vi "DialogCfg.vi"(8 "error in (no error)":errorcluster, 11 "Sequence in":refnum<class "Sequence.lvclass">) -> (0 "error out":errorcluster, 1 "Cancelled?":bool, 3 "Sequence out":refnum<class "Sequence.lvclass">, 4 "TestSequence":T1[](array[typedef]))   [LabVIEW 2017]
uses:
  SequenceSubvis/PolarizationSelect.ctl
  SequenceSubvis/RF Direction.ctl
  Sequence.lvclass
  SequenceSubvis/TestStepTypes.ctl
  SequenceSubvis/TestStep-StepType.ctl
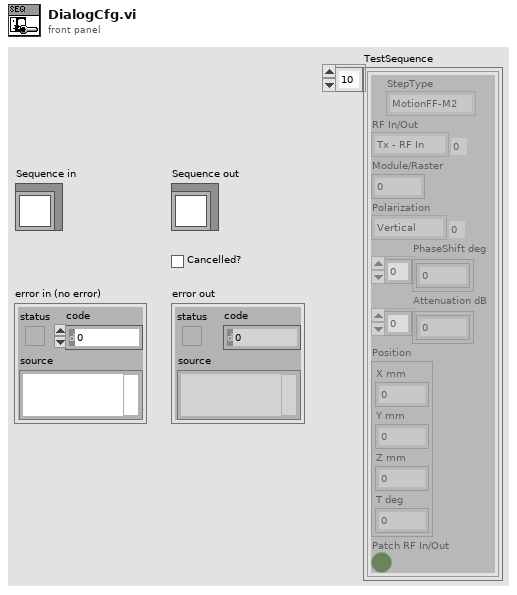
[diagram p1: front panel]
types:
  T1 = typedef "TestStep-StepType.ctl" = cluster{"StepType":T2, "RF In/Out":T3, "Module/Raster":i32, "Polarization":T4, "PhaseShift deg":dbl[], "Attenuation dB":dbl[], "Position":cluster{"X mm":dbl, "Y mm":dbl, "Z mm":dbl, "T deg":dbl}, "Patch RF In/Out":bool}
  T2 = typedef "TestStepTypes.ctl" = enum16{"MotionFF-M2", "Motion", "SweepTest", "RasterTest", "Finish", "64ModuleCfg"}
  T3 = typedef "RF Direction.ctl" = enum16{"Tx - RF In", "Rx - RF Out"}
  T4 = typedef "PolarizationSelect.ctl" = enum16{"Vertical", "Horizontal"}
  T5 = cluster{"StepType":enum16{"Patch", "Motion", "SweepTest", "RasterTest", "Finish"}, "RF In/Out":T3, "Module/Raster":i32, "Polarization":T4, "PhaseShift deg":dbl[], "Attenuation dB":dbl[], "Position":cluster{"X mm":dbl, "Y mm":dbl, "Z mm":dbl, "T deg":dbl}, "Patch RF In/Out":bool}[]
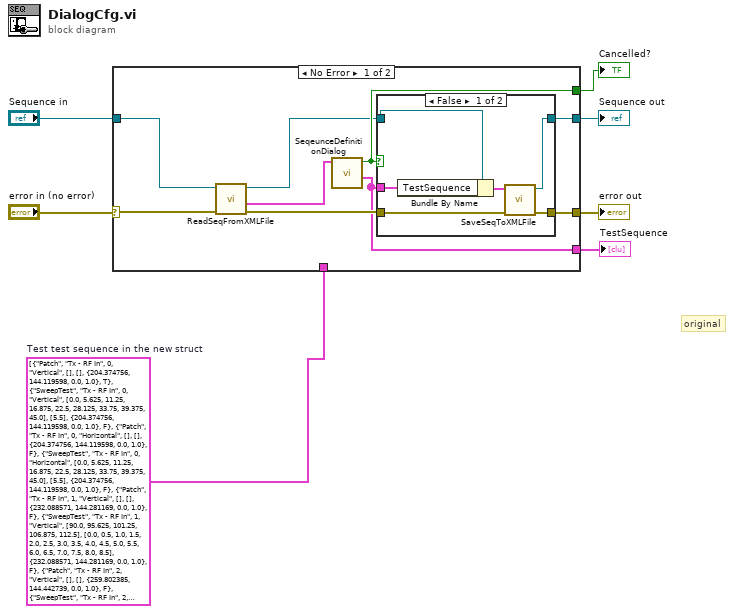
[diagram p0: block diagram]
diagram:
  w1 = T5 [{"StepType"=enum."Patch", "RF In/Out"=enum."Tx - RF In", "Module/Raster"=0, "Polarization"=enum."Vertical", "PhaseShift deg"=[], "Attenuation dB"=[], "Position"={"X mm"=204.374756, "Y mm"=144.119598, "Z mm"=0.0, "T deg"=1.0}, "Patch RF In/Out"=TRUE}, {"StepType"=enum."SweepTest", "RF In/Out"=enum."Tx - RF In", "Module/Raster"=0, "Polarization"=enum."Vertical", "PhaseShift deg"=[0.0, 5.625, 11.25, 16.875, 22.5, 28.125, 33.75, 39.375, 45.0], "Attenuation dB"=[5.5], "Position"={"X mm"=204.374756, "Y mm"=144.119598, "Z mm"=0.0, "T deg"=1.0}, "Patch RF In/Out"=FALSE}, {"StepType"=enum."Patch", "RF In/Out"=enum."Tx - RF In", "Module/Raster"=0, "Polarization"=enum."Horizontal", "PhaseShift deg"=[], "Attenuation dB"=[], "Position"={"X mm"=204.374756, "Y mm"=144.119598, "Z mm"=0.0, "T deg"=1.0}, "Patch RF In/Out"=FALSE}, {"StepType"=enum."SweepTest", "RF In/Out"=enum."Tx - RF In", "Module/Raster"=0, "Polarization"=enum."Horizontal", "PhaseShift deg"=[0.0, 5.625, 11.25, 16.875, 22.5, 28.125, 33.75, 39.375, 45.0], "Attenuation dB"=[5.5], "Position"={"X mm"=204.374756, "Y mm"=144.119598, "Z mm"=0.0, "T deg"=1.0}, "Patch RF In/Out"=FALSE}, {"StepType"=enum."Patch", "RF In/Out"=enum."Tx - RF In", "Module/Raster"=1, "Polarization"=enum."Vertical", "PhaseShift deg"=[], "Attenuation dB"=[], "Position"={"X mm"=232.088571, "Y mm"=144.281169, "Z mm"=0.0, "T deg"=1.0}, "Patch RF In/Out"=FALSE}, {"StepType"=enum."SweepTest", "RF In/Out"=enum."Tx - RF In", "Module/Raster"=1, "Polarization"=enum."Vertical", "PhaseShift deg"=[90.0, 95.625, 101.25, 106.875, 112.5], "Attenuation dB"=[0.0, 0.5, 1.0, 1.5, 2.0, 2.5, 3.0, 3.5, 4.0, 4.5, 5.0, 5.5, 6.0, 6.5, 7.0, 7.5, 8.0, 8.5], "Position"={"X mm"=232.088571, "Y mm"=144.281169, "Z mm"=0.0, "T deg"=1.0}, "Patch RF In/Out"=FALSE}, {"StepType"=enum."Patch", "RF In/Out"=enum."Tx - RF In", "Module/Raster"=2, "Polarization"=enum."Vertical", "PhaseShift deg"=[], "Attenuation dB"=[], "Position"={"X mm"=259.802385, "Y mm"=144.442739, "Z mm"=0.0, "T deg"=1.0}, "Patch RF In/Out"=FALSE}, {"StepType"=enum."SweepTest", "RF In/Out"=enum."Tx - RF In", "Module/Raster"=2, "Polarization"=enum."Vertical", "PhaseShift deg"=[11.25, 16.875, 22.5, 28.125, 33.75, 39.375, 45.0, 50.625, 56.25, 61.875, 67.5, 73.125, 78.75, 84.375, 90.0, 95.625, 101.25, 106.875, 112.5], "Attenuation dB"=[0.0, 5.5, 7.0, 8.0, 9.0, 9.5], "Position"={"X mm"=259.802385, "Y mm"=144.442739, "Z mm"=0.0, "T deg"=1.0}, "Patch RF In/Out"=FALSE}, {"StepType"=enum."Patch", "RF In/Out"=enum."Tx - RF In", "Module/Raster"=15, "Polarization"=enum."Vertical", "PhaseShift deg"=[], "Attenuation dB"=[], "Position"={"X mm"=398.209889, "Y mm"=172.964406, "Z mm"=0.0, "T deg"=1.0}, "Patch RF In/Out"=FALSE}, {"StepType"=enum."SweepTest", "RF In/Out"=enum."Tx - RF In", "Module/Raster"=15, "Polarization"=enum."Vertical", "PhaseShift deg"=[0.0, 5.625, 11.25, 16.875, 22.5], "Attenuation dB"=[0.0, 0.5, 1.0, 1.5, 2.0], "Position"={"X mm"=398.209889, "Y mm"=172.964406, "Z mm"=0.0, "T deg"=1.0}, "Patch RF In/Out"=FALSE}, {"StepType"=enum."Patch", "RF In/Out"=enum."Tx - RF In", "Module/Raster"=17, "Polarization"=enum."Vertical", "PhaseShift deg"=[], "Attenuation dB"=[], "Position"={"X mm"=231.76543, "Y mm"=199.708798, "Z mm"=0.0, "T deg"=1.0}, "Patch RF In/Out"=FALSE}, {"StepType"=enum."SweepTest", "RF In/Out"=enum."Tx - RF In", "Module/Raster"=17, "Polarization"=enum."Vertical", "PhaseShift deg"=[0.0, 5.625], "Attenuation dB"=[0.0, 0.5], "Position"={"X mm"=231.76543, "Y mm"=199.708798, "Z mm"=0.0, "T deg"=1.0}, "Patch RF In/Out"=FALSE}, {"StepType"=enum."Patch", "RF In/Out"=enum."Tx - RF In", "Module/Raster"=21, "Polarization"=enum."Vertical", "PhaseShift deg"=[], "Attenuation dB"=[], "Position"={"X mm"=342.620689, "Y mm"=200.35508, "Z mm"=0.0, "T deg"=1.0}, "Patch RF In/Out"=FALSE}, {"StepType"=enum."SweepTest", "RF In/Out"=enum."Tx - RF In", "Module/Raster"=21, "Polarization"=enum."Vertical", "PhaseShift deg"=[0.0], "Attenuation dB"=[0.0], "Position"={"X mm"=342.620689, "Y mm"=200.35508, "Z mm"=0.0, "T deg"=1.0}, "Patch RF In/Out"=FALSE}, {"StepType"=enum."Patch", "RF In/Out"=enum."Tx - RF In", "Module/Raster"=23, "Polarization"=enum."Vertical", "PhaseShift deg"=[], "Attenuation dB"=[], "Position"={"X mm"=398.048318, "Y mm"=200.678221, "Z mm"=0.0, "T deg"=1.0}, "Patch RF In/Out"=FALSE}, {"StepType"=enum."SweepTest", "RF In/Out"=enum."Tx - RF In", "Module/Raster"=23, "Polarization"=enum."Vertical", "PhaseShift deg"=[0.0], "Attenuation dB"=[0.0], "Position"={"X mm"=398.048318, "Y mm"=200.678221, "Z mm"=0.0, "T deg"=1.0}, "Patch RF In/Out"=FALSE}, {"StepType"=enum."Patch", "RF In/Out"=enum."Tx - RF In", "Module/Raster"=24, "Polarization"=enum."Vertical", "PhaseShift deg"=[], "Attenuation dB"=[], "Position"={"X mm"=203.890045, "Y mm"=227.261043, "Z mm"=0.0, "T deg"=1.0}, "Patch RF In/Out"=FALSE}, {"StepType"=enum."SweepTest", "RF In/Out"=enum."Tx - RF In", "Module/Raster"=24, "Polarization"=enum."Vertical", "PhaseShift deg"=[0.0, 5.625, 11.25], "Attenuation dB"=[0.0], "Position"={"X mm"=203.890045, "Y mm"=227.261043, "Z mm"=0.0, "T deg"=1.0}, "Patch RF In/Out"=FALSE}, {"StepType"=enum."Patch", "RF In/Out"=enum."Tx - RF In", "Module/Raster"=25, "Polarization"=enum."Vertical", "PhaseShift deg"=[], "Attenuation dB"=[], "Position"={"X mm"=231.603859, "Y mm"=227.422613, "Z mm"=0.0, "T deg"=1.0}, "Patch RF In/Out"=FALSE}, {"StepType"=enum."SweepTest", "RF In/Out"=enum."Tx - RF In", "Module/Raster"=25, "Polarization"=enum."Vertical", "PhaseShift deg"=[0.0], "Attenuation dB"=[0.0], "Position"={"X mm"=231.603859, "Y mm"=227.422613, "Z mm"=0.0, "T deg"=1.0}, "Patch RF In/Out"=FALSE}, {"StepType"=enum."Patch", "RF In/Out"=enum."Tx - RF In", "Module/Raster"=31, "Polarization"=enum."Vertical", "PhaseShift deg"=[], "Attenuation dB"=[], "Position"={"X mm"=397.886748, "Y mm"=228.392036, "Z mm"=0.0, "T deg"=1.0}, "Patch RF In/Out"=FALSE}, {"StepType"=enum."SweepTest", "RF In/Out"=enum."Tx - RF In", "Module/Raster"=31, "Polarization"=enum."Vertical", "PhaseShift deg"=[0.0, 5.625], "Attenuation dB"=[0.0], "Position"={"X mm"=397.886748, "Y mm"=228.392036, "Z mm"=0.0, "T deg"=1.0}, "Patch RF In/Out"=FALSE}, {"StepType"=enum."Patch", "RF In/Out"=enum."Tx - RF In", "Module/Raster"=31, "Polarization"=enum."Horizontal", "PhaseShift deg"=[], "Attenuation dB"=[], "Position"={"X mm"=397.886748, "Y mm"=228.392036, "Z mm"=0.0, "T deg"=1.0}, "Patch RF In/Out"=FALSE}, {"StepType"=enum."SweepTest", "RF In/Out"=enum."Tx - RF In", "Module/Raster"=31, "Polarization"=enum."Horizontal", "PhaseShift deg"=[0.0, 5.625], "Attenuation dB"=[0.0], "Position"={"X mm"=397.886748, "Y mm"=228.392036, "Z mm"=0.0, "T deg"=1.0}, "Patch RF In/Out"=FALSE}, {"StepType"=enum."Patch", "RF In/Out"=enum."Tx - RF In", "Module/Raster"=39, "Polarization"=enum."Vertical", "PhaseShift deg"=[], "Attenuation dB"=[], "Position"={"X mm"=397.725177, "Y mm"=256.10585, "Z mm"=0.0, "T deg"=1.0}, "Patch RF In/Out"=FALSE}, {"StepType"=enum."SweepTest", "RF In/Out"=enum."Tx - RF In", "Module/Raster"=39, "Polarization"=enum."Vertical", "PhaseShift deg"=[0.0], "Attenuation dB"=[0.0], "Position"={"X mm"=397.725177, "Y mm"=256.10585, "Z mm"=0.0, "T deg"=1.0}, "Patch RF In/Out"=FALSE}, {"StepType"=enum."Patch", "RF In/Out"=enum."Tx - RF In", "Module/Raster"=44, "Polarization"=enum."Vertical", "PhaseShift deg"=[], "Attenuation dB"=[], "Position"={"X mm"=314.422163, "Y mm"=283.334954, "Z mm"=0.0, "T deg"=1.0}, "Patch RF In/Out"=FALSE}, {"StepType"=enum."SweepTest", "RF In/Out"=enum."Tx - RF In", "Module/Raster"=44, "Polarization"=enum."Vertical", "PhaseShift deg"=[0.0, 5.625], "Attenuation dB"=[0.0, 0.5], "Position"={"X mm"=314.422163, "Y mm"=283.334954, "Z mm"=0.0, "T deg"=1.0}, "Patch RF In/Out"=FALSE}, {"StepType"=enum."Patch", "RF In/Out"=enum."Tx - RF In", "Module/Raster"=45, "Polarization"=enum."Vertical", "PhaseShift deg"=[], "Attenuation dB"=[], "Position"={"X mm"=342.135977, "Y mm"=283.496524, "Z mm"=0.0, "T deg"=1.0}, "Patch RF In/Out"=FALSE}, {"StepType"=enum."SweepTest", "RF In/Out"=enum."Tx - RF In", "Module/Raster"=45, "Polarization"=enum."Vertical", "PhaseShift deg"=[0.0], "Attenuation dB"=[0.0], "Position"={"X mm"=342.135977, "Y mm"=283.496524, "Z mm"=0.0, "T deg"=1.0}, "Patch RF In/Out"=FALSE}, {"StepType"=enum."Patch", "RF In/Out"=enum."Tx - RF In", "Module/Raster"=46, "Polarization"=enum."Vertical", "PhaseShift deg"=[], "Attenuation dB"=[], "Position"={"X mm"=369.849792, "Y mm"=283.658095, "Z mm"=0.0, "T deg"=1.0}, "Patch RF In/Out"=FALSE}, {"StepType"=enum."SweepTest", "RF In/Out"=enum."Tx - RF In", "Module/Raster"=46, "Polarization"=enum."Vertical", "PhaseShift deg"=[0.0, 5.625], "Attenuation dB"=[0.0, 0.5], "Position"={"X mm"=369.849792, "Y mm"=283.658095, "Z mm"=0.0, "T deg"=1.0}, "Patch RF In/Out"=FALSE}, {"StepType"=enum."Patch", "RF In/Out"=enum."Tx - RF In", "Module/Raster"=47, "Polarization"=enum."Vertical", "PhaseShift deg"=[], "Attenuation dB"=[], "Position"={"X mm"=397.563607, "Y mm"=283.819665, "Z mm"=0.0, "T deg"=1.0}, "Patch RF In/Out"=FALSE}, {"StepType"=enum."SweepTest", "RF In/Out"=enum."Tx - RF In", "Module/Raster"=47, "Polarization"=enum."Vertical", "PhaseShift deg"=[0.0], "Attenuation dB"=[0.0], "Position"={"X mm"=397.563607, "Y mm"=283.819665, "Z mm"=0.0, "T deg"=1.0}, "Patch RF In/Out"=FALSE}, {"StepType"=enum."Patch", "RF In/Out"=enum."Tx - RF In", "Module/Raster"=48, "Polarization"=enum."Vertical", "PhaseShift deg"=[], "Attenuation dB"=[], "Position"={"X mm"=203.405333, "Y mm"=310.402487, "Z mm"=0.0, "T deg"=1.0}, "Patch RF In/Out"=FALSE}, {"StepType"=enum."SweepTest", "RF In/Out"=enum."Tx - RF In", "Module/Raster"=48, "Polarization"=enum."Vertical", "PhaseShift deg"=[28.125], "Attenuation dB"=[2.5], "Position"={"X mm"=203.405333, "Y mm"=310.402487, "Z mm"=0.0, "T deg"=1.0}, "Patch RF In/Out"=FALSE}, {"StepType"=enum."Patch", "RF In/Out"=enum."Tx - RF In", "Module/Raster"=48, "Polarization"=enum."Horizontal", "PhaseShift deg"=[], "Attenuation dB"=[], "Position"={"X mm"=203.405333, "Y mm"=310.402487, "Z mm"=0.0, "T deg"=1.0}, "Patch RF In/Out"=FALSE}, {"StepType"=enum."SweepTest", "RF In/Out"=enum."Tx - RF In", "Module/Raster"=48, "Polarization"=enum."Horizontal", "PhaseShift deg"=[28.125], "Attenuation dB"=[2.5], "Position"={"X mm"=203.405333, "Y mm"=310.402487, "Z mm"=0.0, "T deg"=1.0}, "Patch RF In/Out"=FALSE}, {"StepType"=enum."Patch", "RF In/Out"=enum."Tx - RF In", "Module/Raster"=55, "Polarization"=enum."Vertical", "PhaseShift deg"=[], "Attenuation dB"=[], "Position"={"X mm"=397.402037, "Y mm"=311.53348, "Z mm"=0.0, "T deg"=1.0}, "Patch RF In/Out"=FALSE}, {"StepType"=enum."SweepTest", "RF In/Out"=enum."Tx - RF In", "Module/Raster"=55, "Polarization"=enum."Vertical", "PhaseShift deg"=[0.0, 5.625, 11.25, 16.875, 22.5], "Attenuation dB"=[0.0, 0.5, 1.0], "Position"={"X mm"=397.402037, "Y mm"=311.53348, "Z mm"=0.0, "T deg"=1.0}, "Patch RF In/Out"=FALSE}, {"StepType"=enum."Patch", "RF In/Out"=enum."Tx - RF In", "Module/Raster"=59, "Polarization"=enum."Vertical", "PhaseShift deg"=[], "Attenuation dB"=[], "Position"={"X mm"=286.385207, "Y mm"=338.601013, "Z mm"=0.0, "T deg"=1.0}, "Patch RF In/Out"=FALSE}, {"StepType"=enum."SweepTest", "RF In/Out"=enum."Tx - RF In", "Module/Raster"=59, "Polarization"=enum."Vertical", "PhaseShift deg"=[0.0], "Attenuation dB"=[0.0], "Position"={"X mm"=286.385207, "Y mm"=338.601013, "Z mm"=0.0, "T deg"=1.0}, "Patch RF In/Out"=FALSE}, {"StepType"=enum."Patch", "RF In/Out"=enum."Tx - RF In", "Module/Raster"=59, "Polarization"=enum."Horizontal", "PhaseShift deg"=[], "Attenuation dB"=[], "Position"={"X mm"=286.385207, "Y mm"=338.601013, "Z mm"=0.0, "T deg"=1.0}, "Patch RF In/Out"=FALSE}, {"StepType"=enum."SweepTest", "RF In/Out"=enum."Tx - RF In", "Module/Raster"=59, "Polarization"=enum."Horizontal", "PhaseShift deg"=[0.0], "Attenuation dB"=[0.0], "Position"={"X mm"=286.385207, "Y mm"=338.601013, "Z mm"=0.0, "T deg"=1.0}, "Patch RF In/Out"=FALSE}, {"StepType"=enum."Patch", "RF In/Out"=enum."Tx - RF In", "Module/Raster"=62, "Polarization"=enum."Vertical", "PhaseShift deg"=[], "Attenuation dB"=[], "Position"={"X mm"=369.526651, "Y mm"=339.085724, "Z mm"=0.0, "T deg"=1.0}, "Patch RF In/Out"=FALSE}, {"StepType"=enum."SweepTest", "RF In/Out"=enum."Tx - RF In", "Module/Raster"=62, "Polarization"=enum."Vertical", "PhaseShift deg"=[0.0, 5.625, 11.25, 16.875, 22.5, 28.125], "Attenuation dB"=[0.0, 0.5, 1.0, 1.5, 2.0, 2.5], "Position"={"X mm"=369.526651, "Y mm"=339.085724, "Z mm"=0.0, "T deg"=1.0}, "Patch RF In/Out"=FALSE}, {"StepType"=enum."Patch", "RF In/Out"=enum."Tx - RF In", "Module/Raster"=63, "Polarization"=enum."Vertical", "PhaseShift deg"=[], "Attenuation dB"=[], "Position"={"X mm"=397.240466, "Y mm"=339.247295, "Z mm"=0.0, "T deg"=1.0}, "Patch RF In/Out"=FALSE}, {"StepType"=enum."SweepTest", "RF In/Out"=enum."Tx - RF In", "Module/Raster"=63, "Polarization"=enum."Vertical", "PhaseShift deg"=[0.0, 5.625, 11.25, 16.875, 22.5, 28.125], "Attenuation dB"=[0.0, 0.5, 1.0, 1.5, 2.0, 2.5], "Position"={"X mm"=397.240466, "Y mm"=339.247295, "Z mm"=0.0, "T deg"=1.0}, "Patch RF In/Out"=FALSE}, {"StepType"=enum."Patch", "RF In/Out"=enum."Rx - RF Out", "Module/Raster"=0, "Polarization"=enum."Vertical", "PhaseShift deg"=[], "Attenuation dB"=[], "Position"={"X mm"=204.374756, "Y mm"=144.119598, "Z mm"=0.0, "T deg"=1.0}, "Patch RF In/Out"=TRUE}, {"StepType"=enum."SweepTest", "RF In/Out"=enum."Rx - RF Out", "Module/Raster"=0, "Polarization"=enum."Vertical", "PhaseShift deg"=[0.0, 5.625, 11.25, 16.875, 22.5, 28.125, 33.75, 39.375, 45.0], "Attenuation dB"=[5.5], "Position"={"X mm"=204.374756, "Y mm"=144.119598, "Z mm"=0.0, "T deg"=1.0}, "Patch RF In/Out"=FALSE}, {"StepType"=enum."Patch", "RF In/Out"=enum."Rx - RF Out", "Module/Raster"=0, "Polarization"=enum."Horizontal", "PhaseShift deg"=[], "Attenuation dB"=[], "Position"={"X mm"=204.374756, "Y mm"=144.119598, "Z mm"=0.0, "T deg"=1.0}, "Patch RF In/Out"=FALSE}, {"StepType"=enum."SweepTest", "RF In/Out"=enum."Rx - RF Out", "Module/Raster"=0, "Polarization"=enum."Horizontal", "PhaseShift deg"=[0.0, 5.625, 11.25, 16.875, 22.5, 28.125, 33.75, 39.375, 45.0], "Attenuation dB"=[5.5], "Position"={"X mm"=204.374756, "Y mm"=144.119598, "Z mm"=0.0, "T deg"=1.0}, "Patch RF In/Out"=FALSE}, {"StepType"=enum."Patch", "RF In/Out"=enum."Rx - RF Out", "Module/Raster"=17, "Polarization"=enum."Horizontal", "PhaseShift deg"=[], "Attenuation dB"=[], "Position"={"X mm"=231.76543, "Y mm"=199.708798, "Z mm"=0.0, "T deg"=1.0}, "Patch RF In/Out"=FALSE}, {"StepType"=enum."SweepTest", "RF In/Out"=enum."Rx - RF Out", "Module/Raster"=17, "Polarization"=enum."Horizontal", "PhaseShift deg"=[0.0, 5.625], "Attenuation dB"=[0.0, 0.5], "Position"={"X mm"=231.76543, "Y mm"=199.708798, "Z mm"=0.0, "T deg"=1.0}, "Patch RF In/Out"=FALSE}, {"StepType"=enum."Patch", "RF In/Out"=enum."Rx - RF Out", "Module/Raster"=28, "Polarization"=enum."Vertical", "PhaseShift deg"=[], "Attenuation dB"=[], "Position"={"X mm"=314.745304, "Y mm"=227.907324, "Z mm"=0.0, "T deg"=1.0}, "Patch RF In/Out"=FALSE}, {"StepType"=enum."SweepTest", "RF In/Out"=enum."Rx - RF Out", "Module/Raster"=28, "Polarization"=enum."Vertical", "PhaseShift deg"=[0.0], "Attenuation dB"=[0.0], "Position"={"X mm"=314.745304, "Y mm"=227.907324, "Z mm"=0.0, "T deg"=1.0}, "Patch RF In/Out"=FALSE}, {"StepType"=enum."Patch", "RF In/Out"=enum."Rx - RF Out", "Module/Raster"=28, "Polarization"=enum."Horizontal", "PhaseShift deg"=[], "Attenuation dB"=[], "Position"={"X mm"=314.745304, "Y mm"=227.907324, "Z mm"=0.0, "T deg"=1.0}, "Patch RF In/Out"=FALSE}, {"StepType"=enum."SweepTest", "RF In/Out"=enum."Rx - RF Out", "Module/Raster"=28, "Polarization"=enum."Horizontal", "PhaseShift deg"=[0.0], "Attenuation dB"=[0.0], "Position"={"X mm"=314.745304, "Y mm"=227.907324, "Z mm"=0.0, "T deg"=1.0}, "Patch RF In/Out"=FALSE}, {"StepType"=enum."Patch", "RF In/Out"=enum."Rx - RF Out", "Module/Raster"=31, "Polarization"=enum."Vertical", "PhaseShift deg"=[], "Attenuation dB"=[], "Position"={"X mm"=397.886748, "Y mm"=228.392036, "Z mm"=0.0, "T deg"=1.0}, "Patch RF In/Out"=FALSE}, {"StepType"=enum."SweepTest", "RF In/Out"=enum."Rx - RF Out", "Module/Raster"=31, "Polarization"=enum."Vertical", "PhaseShift deg"=[0.0, 5.625], "Attenuation dB"=[0.0], "Position"={"X mm"=397.886748, "Y mm"=228.392036, "Z mm"=0.0, "T deg"=1.0}, "Patch RF In/Out"=FALSE}, {"StepType"=enum."Patch", "RF In/Out"=enum."Rx - RF Out", "Module/Raster"=31, "Polarization"=enum."Horizontal", "PhaseShift deg"=[], "Attenuation dB"=[], "Position"={"X mm"=397.886748, "Y mm"=228.392036, "Z mm"=0.0, "T deg"=1.0}, "Patch RF In/Out"=FALSE}, {"StepType"=enum."SweepTest", "RF In/Out"=enum."Rx - RF Out", "Module/Raster"=31, "Polarization"=enum."Horizontal", "PhaseShift deg"=[0.0, 5.625], "Attenuation dB"=[0.0], "Position"={"X mm"=397.886748, "Y mm"=228.392036, "Z mm"=0.0, "T deg"=1.0}, "Patch RF In/Out"=FALSE}, {"StepType"=enum."Patch", "RF In/Out"=enum."Rx - RF Out", "Module/Raster"=36, "Polarization"=enum."Vertical", "PhaseShift deg"=[], "Attenuation dB"=[], "Position"={"X mm"=314.583733, "Y mm"=255.621139, "Z mm"=0.0, "T deg"=1.0}, "Patch RF In/Out"=FALSE}, {"StepType"=enum."SweepTest", "RF In/Out"=enum."Rx - RF Out", "Module/Raster"=36, "Polarization"=enum."Vertical", "PhaseShift deg"=[28.125, 33.75, 39.375, 45.0, 50.625], "Attenuation dB"=[5.0, 5.5, 6.0, 6.5, 7.0], "Position"={"X mm"=314.583733, "Y mm"=255.621139, "Z mm"=0.0, "T deg"=1.0}, "Patch RF In/Out"=FALSE}, {"StepType"=enum."Patch", "RF In/Out"=enum."Rx - RF Out", "Module/Raster"=36, "Polarization"=enum."Horizontal", "PhaseShift deg"=[], "Attenuation dB"=[], "Position"={"X mm"=314.583733, "Y mm"=255.621139, "Z mm"=0.0, "T deg"=1.0}, "Patch RF In/Out"=FALSE}, {"StepType"=enum."SweepTest", "RF In/Out"=enum."Rx - RF Out", "Module/Raster"=36, "Polarization"=enum."Horizontal", "PhaseShift deg"=[28.125, 33.75, 39.375, 45.0, 50.625], "Attenuation dB"=[5.0, 5.5, 6.0, 6.5, 7.0], "Position"={"X mm"=314.583733, "Y mm"=255.621139, "Z mm"=0.0, "T deg"=1.0}, "Patch RF In/Out"=FALSE}, {"StepType"=enum."Patch", "RF In/Out"=enum."Rx - RF Out", "Module/Raster"=48, "Polarization"=enum."Vertical", "PhaseShift deg"=[], "Attenuation dB"=[], "Position"={"X mm"=203.405333, "Y mm"=310.402487, "Z mm"=0.0, "T deg"=1.0}, "Patch RF In/Out"=FALSE}, {"StepType"=enum."SweepTest", "RF In/Out"=enum."Rx - RF Out", "Module/Raster"=48, "Polarization"=enum."Vertical", "PhaseShift deg"=[28.125], "Attenuation dB"=[2.5], "Position"={"X mm"=203.405333, "Y mm"=310.402487, "Z mm"=0.0, "T deg"=1.0}, "Patch RF In/Out"=FALSE}, {"StepType"=enum."Patch", "RF In/Out"=enum."Rx - RF Out", "Module/Raster"=48, "Polarization"=enum."Horizontal", "PhaseShift deg"=[], "Attenuation dB"=[], "Position"={"X mm"=203.405333, "Y mm"=310.402487, "Z mm"=0.0, "T deg"=1.0}, "Patch RF In/Out"=FALSE}, {"StepType"=enum."SweepTest", "RF In/Out"=enum."Rx - RF Out", "Module/Raster"=48, "Polarization"=enum."Horizontal", "PhaseShift deg"=[28.125], "Attenuation dB"=[2.5], "Position"={"X mm"=203.405333, "Y mm"=310.402487, "Z mm"=0.0, "T deg"=1.0}, "Patch RF In/Out"=FALSE}, {"StepType"=enum."Patch", "RF In/Out"=enum."Rx - RF Out", "Module/Raster"=59, "Polarization"=enum."Vertical", "PhaseShift deg"=[], "Attenuation dB"=[], "Position"={"X mm"=286.385207, "Y mm"=338.601013, "Z mm"=0.0, "T deg"=1.0}, "Patch RF In/Out"=FALSE}, {"StepType"=enum."SweepTest", "RF In/Out"=enum."Rx - RF Out", "Module/Raster"=59, "Polarization"=enum."Vertical", "PhaseShift deg"=[0.0], "Attenuation dB"=[0.0], "Position"={"X mm"=286.385207, "Y mm"=338.601013, "Z mm"=0.0, "T deg"=1.0}, "Patch RF In/Out"=FALSE}, {"StepType"=enum."Patch", "RF In/Out"=enum."Rx - RF Out", "Module/Raster"=59, "Polarization"=enum."Horizontal", "PhaseShift deg"=[], "Attenuation dB"=[], "Position"={"X mm"=286.385207, "Y mm"=338.601013, "Z mm"=0.0, "T deg"=1.0}, "Patch RF In/Out"=FALSE}, {"StepType"=enum."SweepTest", "RF In/Out"=enum."Rx - RF Out", "Module/Raster"=59, "Polarization"=enum."Horizontal", "PhaseShift deg"=[0.0], "Attenuation dB"=[0.0], "Position"={"X mm"=286.385207, "Y mm"=338.601013, "Z mm"=0.0, "T deg"=1.0}, "Patch RF In/Out"=FALSE}, {"StepType"=enum."Patch", "RF In/Out"=enum."Rx - RF Out", "Module/Raster"=62, "Polarization"=enum."Vertical", "PhaseShift deg"=[], "Attenuation dB"=[], "Position"={"X mm"=369.526651, "Y mm"=339.085724, "Z mm"=0.0, "T deg"=1.0}, "Patch RF In/Out"=FALSE}, {"StepType"=enum."SweepTest", "RF In/Out"=enum."Rx - RF Out", "Module/Raster"=62, "Polarization"=enum."Vertical", "PhaseShift deg"=[0.0, 5.625, 11.25, 16.875, 22.5, 28.125], "Attenuation dB"=[0.0, 0.5, 1.0, 1.5, 2.0, 2.5], "Position"={"X mm"=369.526651, "Y mm"=339.085724, "Z mm"=0.0, "T deg"=1.0}, "Patch RF In/Out"=FALSE}, {"StepType"=enum."Patch", "RF In/Out"=enum."Rx - RF Out", "Module/Raster"=63, "Polarization"=enum."Vertical", "PhaseShift deg"=[], "Attenuation dB"=[], "Position"={"X mm"=397.240466, "Y mm"=339.247295, "Z mm"=0.0, "T deg"=1.0}, "Patch RF In/Out"=FALSE}, {"StepType"=enum."SweepTest", "RF In/Out"=enum."Rx - RF Out", "Module/Raster"=63, "Polarization"=enum."Vertical", "PhaseShift deg"=[0.0, 5.625, 11.25, 16.875, 22.5, 28.125], "Attenuation dB"=[0.0, 0.5, 1.0, 1.5, 2.0, 2.5], "Position"={"X mm"=397.240466, "Y mm"=339.247295, "Z mm"=0.0, "T deg"=1.0}, "Patch RF In/Out"=FALSE}, {"StepType"=enum."Finish", "RF In/Out"=enum."Tx - RF In", "Module/Raster"=0, "Polarization"=enum."Vertical", "PhaseShift deg"=[], "Attenuation dB"=[], "Position"={"X mm"=204.374756, "Y mm"=144.119598, "Z mm"=0.0, "T deg"=1.0}, "Patch RF In/Out"=FALSE}]  # Test test sequence in the new struct
  # "original"
  n1 = case shown="No Error" "error in (no error)" {
    selector: "error in (no error)" -> [w13 w26]
    tunnel: [w15 w26] -> w6
    tunnel: [w16 w25] -> w4
    tunnel: "Sequence in" -> [w11 w25]
    tunnel: [w14 _] -> w3
    tunnel: [w9 _] -> w2
    tunnel: w1 -> [_ _]
    frame No Error {
      n2 = call "ReadSeqFromXMLFile.vi"("error in (no error)"=w13, "Sequence in"=w11) -> ("error out"=w12:errorcluster, "TestSequence"=w8:T1[], "Sequence out"=w10:refnum<class "Sequence.lvclass">)  [unwired: 5 in, 2 out]
      n3 = call "SeqeunceDefinitionDialog.vi"("TestSequence"=w8) -> ("TestSequence out"=w9:T1[], "Cancelled?"=w14:bool)  [unwired: 9 in]
      n4 = case shown="False" w14 {
        tunnel: [w19 w24] -> w16
        tunnel: w10 -> [w22 w24]
        tunnel: w9 -> [w21 _]
        tunnel: [w18 w23] -> w15
        tunnel: w12 -> [w17 w23]
        frame False {
          n5 = Bundle By Name(cluster=w22, "TestSequence"=w21) -> (w20:cluster{})
          n6 = call "SaveSeqToXMLFile.vi"("error in (no error)"=w17, "Sequence in"=w20) -> ("error out"=w18:errorcluster, "Sequence out"=w19:refnum<class "Sequence.lvclass">)  [unwired: 8 in]
        }
        frame True {
        }
      }
    }
    frame Error {
    }
  }
  "error out" <- w6
  "Sequence out" <- w4
  "Cancelled?" <- w3
  "TestSequence" <- w2
